vi "FTW-Ether-NewLoggerSubscription.vi"(5 "Logger Publisher":string, 11 "error in":errorcluster) -> (4 "Event Logger Subscription":refnum<class "FTW-Subscriber.lvclass">, 15 "error out":errorcluster)   [LabVIEW 2013, in "FTW-Ether.lvclass"]
uses:
  FTW-Ether.lvclass
  Subscriber/FTW-Subscriber.lvclass
  FTW-Ether-Instance.vi
panel:
  # "Inputs"
  # "Outputs"
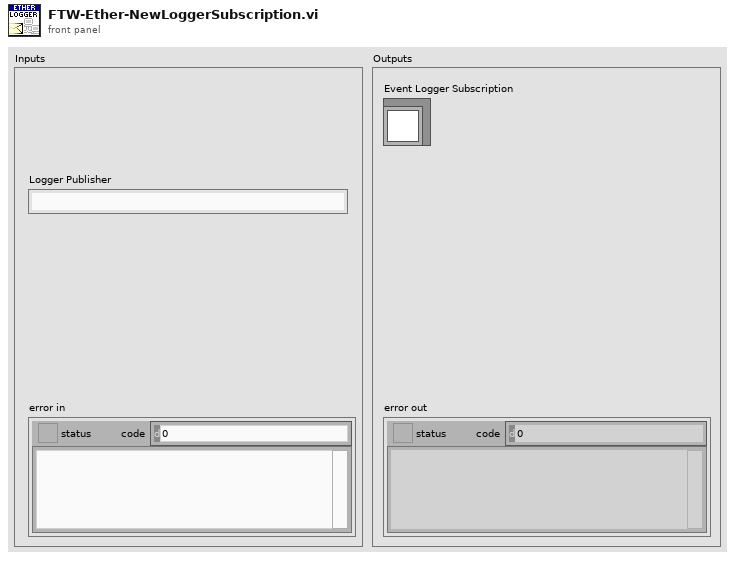
[diagram p1: front panel]
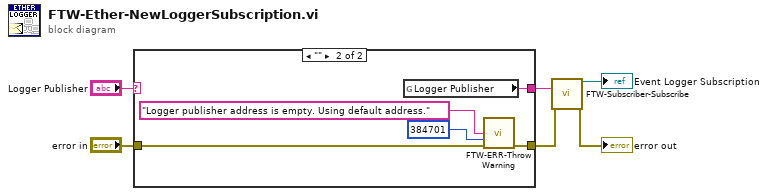
[diagram p0: block diagram]
diagram:
  n1 = case shown="\"\"" "Logger Publisher" {
    selector: "Logger Publisher" -> [w8 _]
    tunnel: [w8 w13] -> w4
    tunnel: "error in" -> [w7 w12]
    tunnel: [w7 w11] -> w1
    frame Default {
    }
    frame "" {
      n2 = global read "FTW-Ether-Instance.vi" "Logger Publisher"() -> (w13:string)
      n3 = call "FTW-ERR-ThrowWarning.vi"("Warning Message"="Logger publisher address is empty. Using default address.", "Error Code"=384701, "error in"=w12) -> ("error out"=w11:errorcluster)  [unwired: 12 in]
    }
  }
  n4 = call "FTW-Subscriber-Subscribe.vi"("Addresses"=w4, "error in"=w1) -> ("FTW-Subscription Out"=→"Event Logger Subscription":refnum<class "FTW-Subscriber.lvclass">, "error out"=→"error out":errorcluster)  [unwired: 11 in, 1 out]
